vi "TestLog.Initial.vi"(8 "错误输入（无错误）":errorcluster, 11 "TestLog_Record_Name":string) -> (0 "错误输出":errorcluster, 1 "New？":bool, 2 "OK?":bool, 3 "TestLog_Recorder":refnum<queue>)   [LabVIEW 2012, in "Lib_UEL.ATE.lvlib" / "Lib_Report.lvlib"]
uses:
  Lib_Report.lvlib
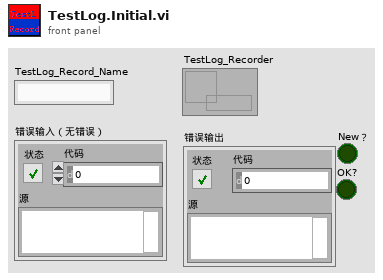
[diagram p1: front panel]
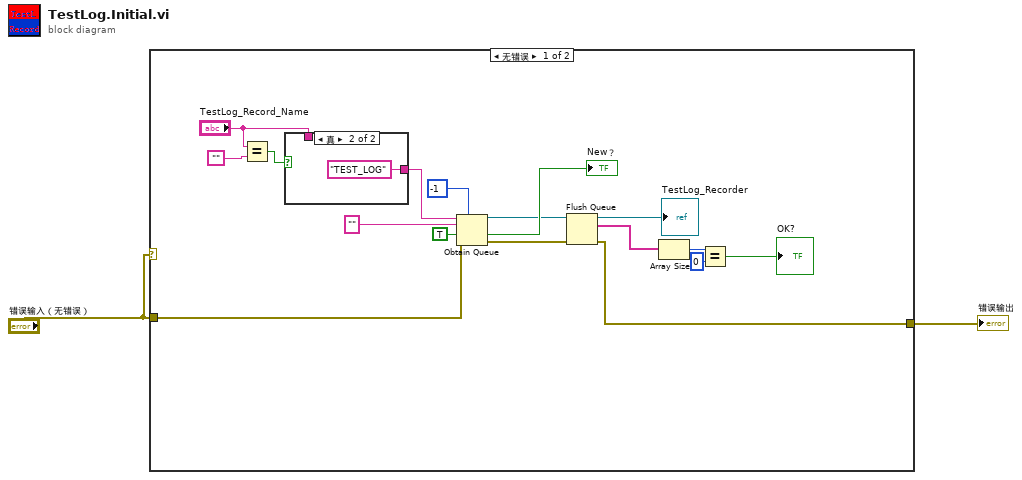
[diagram p0: block diagram]
diagram:
  n1 = case shown="无错误" "错误输入（无错误）" {
    tunnel: "错误输入（无错误）" -> [w17 w22]
    tunnel: [w13 w22] -> w2
    frame No Error {
      n2 = Equal?(x="TestLog_Record_Name", y="") -> (x = y?=w6:bool)
      n3 = case shown="真" w6 {
        tunnel: [w20 "TEST_LOG" ("TestLog_Record_Name")] -> w4
        tunnel: "TestLog_Record_Name" -> [w20 _]
        frame False {
        }
        frame True {
        }
      }
      n4 = Obtain Queue(max queue size (-1, unlimited)=-1 ("队列最大值（-1，无限）"), name (unnamed)=w4, element data type="", create if not found? (T)=TRUE ("如未找到是否创建？(T)"), error in (no error)=w17) -> (queue out=w15:refnum<queue>, created new?=→"New？":bool, error out=w14:errorcluster)
      n5 = Flush Queue(queue=w15, error in (no error)=w14) -> (queue out=→"TestLog_Recorder":refnum<queue>, remaining elements=w11:string[], error out=w13:errorcluster)
      n6 = Array Size(array=w11) -> (size(s)=w10:i32)
      n7 = Equal?(x=w10, y=0) -> (x = y?=→"OK?":bool)
    }
    frame Error {
    }
  }
  "错误输出" <- w2
